vi "Robot Main.vi"() -> ()   [LabVIEW 2017]
doc: "This VI implements the framework and scheduler for your robotics program. It should not be necessary to modify the framework. You are expected to add your code to the VIs called from Robot Main - the ones located in the Team Code folder within the project."
uses:
  <vilib>/Rock Robotics/WPI/Camera/WPI_CameraImageSize.ctl
  Robot Global Data.vi
panel:
  in  "Image Size":T1=enum."320x240"
  in  "Enable Vision":bool
  in  "Finish":bool
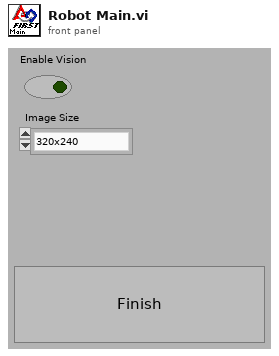
[diagram p1: front panel]
types:
  T1 = typedef "WPI_CameraImageSize.ctl" = enum16{"640x480", "320x240", "160x120", "Custom"}
  T2 = typedef "def HARDWARE CTRL info.ctl" = cluster{"DRIVE MOTORS":T3[], "Controller":T6[], "ENCODERS":T8[], "GYRO HARDWARE":T11, "AIR":cluster{"PRESSURE":T14[], "COMPRESSOR":T16, "SOLENOIDS":T17[]}, "MOTORS":T3[], "SERVOS":T20[], "SONAR":T21[], "RELAY":T24[], "LIMIT":T28[]}
  T3 = typedef "def MOTOR info.ctl" = cluster{"Descr":string, "Motor Controller":T4, "PWM ch":T5, "Invert?":bool, "Installed?":bool, "RefName":string, "stack name":string, "remove deadband":bool}
  T4 = typedef "ctrl MOTOR CTRLR SELECT.ctl" = u16
  T5 = typedef "FPGA_DIOPWMChannel.ctl" = enum8{"PWM 0", "PWM 1", "PWM 2", "PWM 3", "PWM 4", "PWM 5", "PWM 6", "PWM 7", "PWM 8", "PWM 9", "PWM MXP 0", "PWM MXP 1", "PWM MXP 2", "PWM MXP 3", "PWM MXP 4", "PWM MXP 5", "PWM MXP 6", "PWM MXP 7", "PWM MXP 8", "PWM MXP 9", "Invalid"}
  T6 = typedef "def USER CONTROL info.ctl" = cluster{"Descr":string, "Installed?":bool, "RefName":string, "JoystickDevice":T7, "Invert Y axis":bool, "Scale":dbl, "AXIS":string, "BUTTONS":string, "POV":string}
  T7 = typedef "WPI_JoystickDeviceEnum.ctl" = enum16{"USB 0", "USB 1", "USB 2", "USB 3", "USB 4", "USB 5"}
  T8 = typedef "def ENCODER info.ctl" = cluster{"Descr":string, "Installed?":bool, "A Channel":T9, "B Channel":T9, "Invert Direction":bool, "Enum":T10, "Gear ratio":dbl, "Cycles per Rev":dbl, "Diameter (in)":dbl[unit], "RefName":string, "stack name":string, "min rate (hz)":dbl, "Samples":u8, "STACK subnames":cluster{"RESET name":string, "STOPPED name":string, "DIRECTION name":string, "RATE name":string, "INSTALLED name":string}}
  T9 = typedef "FPGA_DIOChannel.ctl" = enum8{"DIO 0", "DIO 1", "DIO 2", "DIO 3", "DIO 4", "DIO 5", "DIO 6", "DIO 7", "DIO 8", "DIO 9", "DIO MXP 0", "DIO MXP 1", "DIO MXP 2", "DIO MXP 3", "DIO MXP 4", "DIO MXP 5", "DIO MXP 6", "DIO MXP 7", "DIO MXP 8", "DIO MXP 9", "DIO MXP 10", "DIO MXP 11", "DIO MXP 12", "DIO MXP 13", "DIO MXP 14", "DIO MXP 15", "SPI Port CS1", "SPI Port CS2", "SPI Port CS3", "SPI Port MISO", "SPI Port MOSI", "Invalid"}
  T10 = typedef "WPI_EncoderType.ctl" = enum16{"1x", "2x", "4x"}
  T11 = typedef "def GYRO info.ctl" = cluster{"Descr":string, "Installed?":bool, "SPI Bus":T12, "AnalogChannel":T13, "Calibrate On Open":bool, "Calibrated Center Voltage":dbl, "Calibration Time (s)":dbl, "Sample Rate (Hz)":dbl, "RefName":string, "stack name":string}
  T12 = typedef "spi_bus.ctl" = enum16{"SPI On-Board, CS0", "SPI On-Board, CS1", "SPI On-Board, CS2", "SPI On-Board, CS3", "SPI MXP", "Invalid"}
  T13 = typedef "ctrl ANALOG CHANNEL SELECT.ctl" = enum8{"AI 0", "AI 1", "Invalid"}
  T14 = typedef "def AIR PRESSURE info.ctl" = cluster{"Descr":string, "Installed?":bool, "Channel":T15, "RefName":string, "stack name":string, "MULTIPLIER":dbl, "OFFSET":dbl, "nominal value":dbl, "warning LOW":dbl, "warning HIGH":dbl}
  T15 = typedef "FPGA_AIChannel.ctl" = enum8{"AI 0", "AI 1", "AI 2", "AI 3", "AI MXP 0", "AI MXP 1", "AI MXP 2", "AI MXP 3", "Invalid"}
  T16 = typedef "def COMPRESSOR info.ctl" = cluster{"Descr":string, "Installed?":bool, "Pneumatics Control Module":u8, "RefName":string, "stack name":string}
  T17 = typedef "def SOLENOID info.ctl" = cluster{"Descr":string, "Installed?":bool, "Pneumatics Control Module (0)":u8, "DBL":bool, "SolenoidChannel":T18, "SolenoidChannel":T18, "Default SET":T19, "RefName":string, "Value":string}
  T18 = typedef "WPI_SolenoidChannel.ctl" = enum8{"Solenoid 0", "Solenoid 1", "Solenoid 2", "Solenoid 3", "Solenoid 4", "Solenoid 5", "Solenoid 6", "Solenoid 7", "Invalid"}
  T19 = typedef "WPI_SolenoidValue.ctl" = enum16{"Off", "On", "Forward", "Reverse"}
  T20 = typedef "def SERVO info.ctl" = cluster{"Descr":string, "PWM ch":T5, "Installed?":bool, "Angular range":dbl, "RefName":string, "stack name":string}
  T21 = typedef "def SONAR info.ctl" = cluster{"Descr":string, "Installed?":bool, "Device type":T22, "PING Channel":T9, "ECHO Channel":T9, "RefName":string, "stack name":string, "Samples":i32, "Range Units":T23}
  T22 = typedef "ctrl SONAR DEVICE SELECT.ctl" = enum16{"SRF04 Digital", "MB1010 Digital", "MB1010 Analog", "SRF08 Digital"}
  T23 = typedef "WPI_UltrasonicRangeUnits.ctl" = enum16{"inches", "mm"}
  T24 = typedef "def RELAY info.ctl" = cluster{"Descr":string, "Installed?":bool, "RelayChannel":T25, "Relay Direction":T26, "Relay Value":T27, "RefName":string, "Value":string}
  T25 = typedef "FPGA_DIORelayChannel.ctl" = enum8{"Relay 0", "Relay 1", "Relay 2", "Relay 3", "Invalid"}
  T26 = typedef "WPI_RelayDirection.ctl" = enum16{"Both directions", "Forward only", "Reverse only"}
  T27 = typedef "WPI_RelayValue.ctl" = enum16{"Off", "On", "Forward", "Reverse"}
  T28 = typedef "def LIMIT SWITCH info.ctl" = cluster{"Descr":string, "Installed?":bool, "A Channel":T9, "Normally Closed?":bool, "RefName":string, "stack name":string}
  T29 = typedef "WPI_DriverStationMatch Info.ctl" = cluster{"Autonomous Elapsed Seconds":dbl, "TeleOp Elapsed Seconds":dbl, "Disabled Elapsed Seconds":dbl, "Visited Autonomous":bool, "Visited TeleOp":bool, "Visited Disabled":bool, "Autonomous Settings":cluster{"Autonomous Style":enum16{"Iterative", "Independent"}, "VI Refnum":refnum<vi>}}
  T30 = typedef "WPI_DriverStationDerivedRobotMode.ctl" = enum16{"Init", "Execute", "Stop"}
  T31 = typedef "WPI_DriverStationRobotMode2.ctl" = enum16{"Autonomous Disabled", "Autonomous Enabled", "Teleop Disabled", "Teleop Enabled", "Disconnected", "Finish", "Test Disabled", "Test Enabled", "Emergency Stopped"}
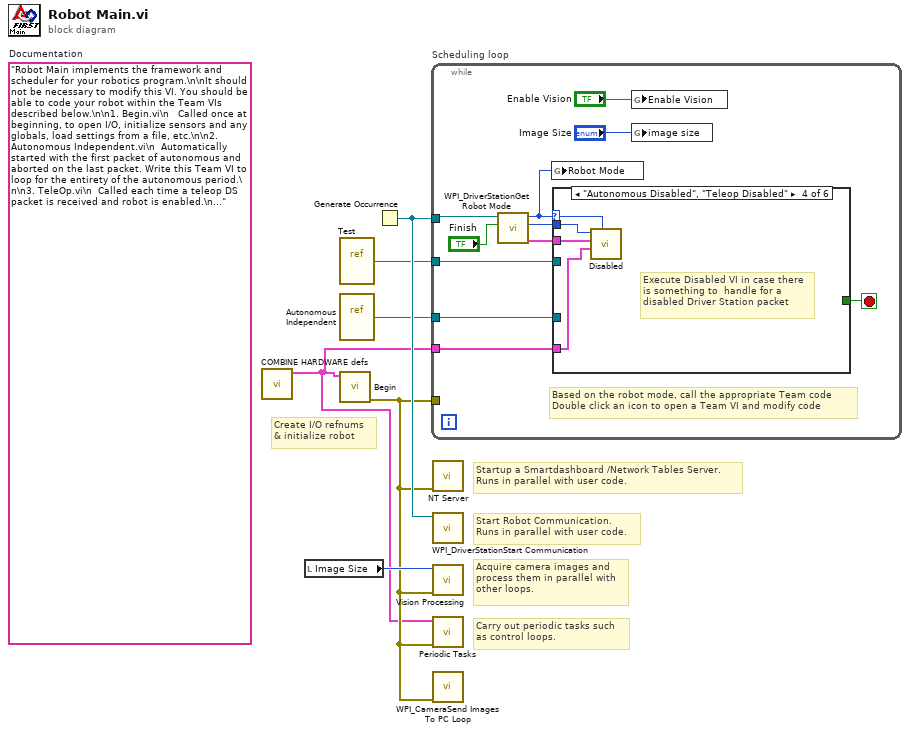
[diagram p0: block diagram]
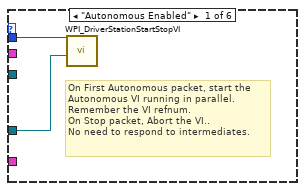
[diagram p2: hidden frame]
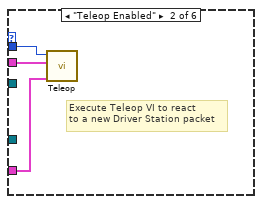
[diagram p3: hidden frame]
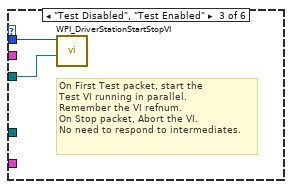
[diagram p4: hidden frame]
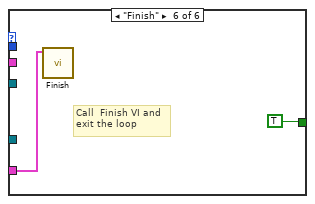
[diagram p6: hidden frame]
diagram:
  (unwired) "Robot Main implements the framework and scheduler for your robotics program.\n\nIt should not be necessary to modify this VI. You should be able to code your robot within the Team VIs described below.\n\n1. Begin.vi\n   Called once at beginning, to open I/O, initialize sensors and any globals, load settings from a file, etc.\n\n2. Autonomous Independent.vi\n  Automatically started with the first packet of autonomous and aborted on the last packet. Write this Team VI to loop for the entirety of the autonomous period.\n\n3. TeleOp.vi\n  Called each time a teleop DS packet is received and robot is enabled.\n\n4. Disabled.vi\n  Called each time a packet is received and the robot is disabled.\n\n5. Test.vi\n  Called Automatically started with the first test packet and aborted on the last. Modify this VI to carry out robot and sensor validation tests.\n\n6. Vision.vi\n  A parallel loop that acquires and processes camera images.\n\n7. PeriodicTasks.vi\n  Parallel loops running at user-defined rates.\n\n8. Finish.vi\n  Called before exiting, so you can save data, clean up I/O, etc.\n"  # Documentation
  # "Startup a Smartdashboard /Network Tables Server.\nRuns in parallel with user code."
  # "Carry out periodic tasks such\nas control loops."
  # "Acquire camera images and\nprocess them in parallel with\nother loops."
  # "Create I/O refnums\n& initialize robot"
  # "Start Robot Communication.\nRuns in parallel with user code."
  n1 = call "COMBINE HARDWARE defs.vi"() -> ("HARDWARE out"=w1:T2)  [unwired: 10 in, 1 out]
  n2 = local read "Image Size"() -> (w3:T1)
  n3 = vi-ref "Test.vi"() -> (w4:refnum<vi>)
  n4 = vi-ref "Autonomous Independent.vi"() -> (w5:refnum<vi>)
  n5 = call "Begin.vi"("HARDWARE cluster"=w1) -> ("error out"=w2:errorcluster)  [unwired: 1 in, 9 out]
  n6 = Generate Occurrence() -> (w6:refnum<k4>)
  n7 = while "Scheduling loop" {
    tunnel: w6 -> [w16]
    tunnel: w2 -> [_]
    tunnel: w5 -> [w11]
    tunnel: w4 -> [w9]
    tunnel: w1 -> [w7]
    stop <- w13 stop-if-true
    # "Based on the robot mode, call the appropriate Team code\nDouble click an icon to open a Team VI and modify code"
    n8 = call <vilib>:"WPI_DriverStationGet Robot Mode.vi"("Finish"="Finish", "DS Occurrence"=w16) -> ("Match Info out"=w14:T29, "Call Context"=w17:T30, "Robot Mode"=w8:T31)  [unwired: 7 out]
    n9 = global write "Robot Global Data.vi" "Robot Mode"(w8) -> ()
    n10 = case shown="\"Autonomous Disabled\", \"Teleop Disabled\"" w8 {
      selector: w8 -> [_ _ _ w26 _ _]
      tunnel: w17 -> [w19 w22 w24 w28 _ _]
      tunnel: w14 -> [_ w21 _ w27 _ _]
      tunnel: [_ _ _ _ _ TRUE] -> w13
      tunnel: w11 -> [w18 _ _ _ _ _]
      tunnel: w9 -> [_ _ w23 _ _ _]
      tunnel: w7 -> [_ w20 _ w25 _ w29]
      frame "Autonomous Enabled" {
        # "On First Autonomous packet, start the\nAutonomous VI running in parallel.\nRemember the VI refnum.\nOn Stop packet, Abort the VI..\nNo need to respond to intermediates."
        n11 = call <vilib>:"WPI_DriverStationStartStopVI.vi"("VI in"=w18, "Call Context"=w19) -> ()  [unwired: 10 in]
      }
      frame "Teleop Enabled" {
        # "Execute Teleop VI to react\nto a new Driver Station packet"
        n12 = call "Teleop.vi"("HARDWARE cluster"=w20, "Match Info"=w21, "Call Context"=w22) -> ()  [unwired: 1 in, 8 out]
      }
      frame "Test Disabled", "Test Enabled" {
        # "On First Test packet, start the\nTest VI running in parallel.\nRemember the VI refnum.\nOn Stop packet, Abort the VI.\nNo need to respond to intermediates."
        n13 = call <vilib>:"WPI_DriverStationStartStopVI.vi"("VI in"=w23, "Call Context"=w24) -> ()  [unwired: 10 in]
      }
      frame "Autonomous Disabled", "Teleop Disabled" {
        # "Execute Disabled VI in case there\nis something to  handle for a\ndisabled Driver Station packet"
        n14 = call "Disabled.vi"("Robot Mode"=w26, "HARDWARE cluster"=w25, "Match Info"=w27, "Call Context"=w28) -> ()  [unwired: 8 out]
      }
      frame "Disconnected", Default {
        # "Driver Station packet didn't arrive.\nPossibly useful for diagnostics"
      }
      frame "Finish" {
        # "Call  Finish VI and\nexit the loop"
        n15 = call "Finish.vi"("HARDWARE cluster"=w29) -> ()  [unwired: 7 out]
      }
    }
    n16 = global write "Robot Global Data.vi" "Enable Vision"("Enable Vision") -> ()
    n17 = global write "Robot Global Data.vi" "image size"("Image Size") -> ()
  }
  n18 = call <vilib>:"NT Server.vi"("error in (no error)"=w2) -> ()  [unwired: 11 in]
  n19 = call <vilib>:"WPI_DriverStationStart Communication.vi"("occurrence"=w6) -> ()  [unwired: 1 in, 10 out]
  n20 = call "Vision Processing.vi"("error in (no error)"=w2, "Image Size"=w3) -> ()  [unwired: 6 out]
  n21 = call "Periodic Tasks.vi"("error in"=w2, "HARDWARE cluster"=w1) -> ()  [unwired: 10 out]
  n22 = call <vilib>:"WPI_CameraSend Images To PC Loop.vi"("error in (no error)"=w2) -> ()  [unwired: 11 in]
